vi "GetPodsStateData.vi"(11 "All Pods In":T17(array[cluster])) -> (2 "All Pod State Data":T18(array[cluster]), 3 "All Pods out":T17(array[cluster]))   [LabVIEW 2014]
uses:
  <vilib>/Rock Robotics/WPI/MotorControl/WPI_MotorControlDeviceRef.ctl
  <vilib>/Rock Robotics/WPI/MotorControl/WPI_MotorControlType.ctl
  <vilib>/Rock Robotics/SystemInterfaces/Typedef/FPGA_TypedefDigitalModule.ctl
  <vilib>/Rock Robotics/SystemInterfaces/DIO/FPGA_DIOPWMChannel.ctl
  <vilib>/Rock Robotics/WPI/PWM/WPI_PWMDeadband.ctl
  <vilib>/Rock Robotics/WPI/CAN/Jaguar/SubVIs/WPI_CANJaguar_ControlMode.ctl
  <vilib>/Rock Robotics/WPI/CAN/TalonSRX/WPI_CANTalonSRX_APIControlMode.ctl
  <vilib>/Rock Robotics/WPI/PWM/WPI_PWMTransform_ConPane.ctl
  <vilib>/Rock Robotics/WPI/AnalogChannel/WPI_AnalogChannelDevRef.ctl
  <vilib>/Rock Robotics/SystemInterfaces/Typedef/FPGA_TypedefAnalogModule.ctl
  <vilib>/Rock Robotics/SystemInterfaces/AI/FPGA_AIChannel.ctl
  <vilib>/Rock Robotics/WPI/Encoder/WPI_EncoderDevRef.ctl
  <vilib>/Rock Robotics/SystemInterfaces/Encoder/FPGA_EncoderIdx.ctl
  <vilib>/Rock Robotics/SystemInterfaces/Counter/FPGA_CounterCtrSystemIndex.ctl
  <vilib>/Rock Robotics/WPI/Encoder/WPI_EncoderType.ctl
  <vilib>/Rock Robotics/SystemInterfaces/Utilities/FPGA_UtilitiesRead LocalTime.vi
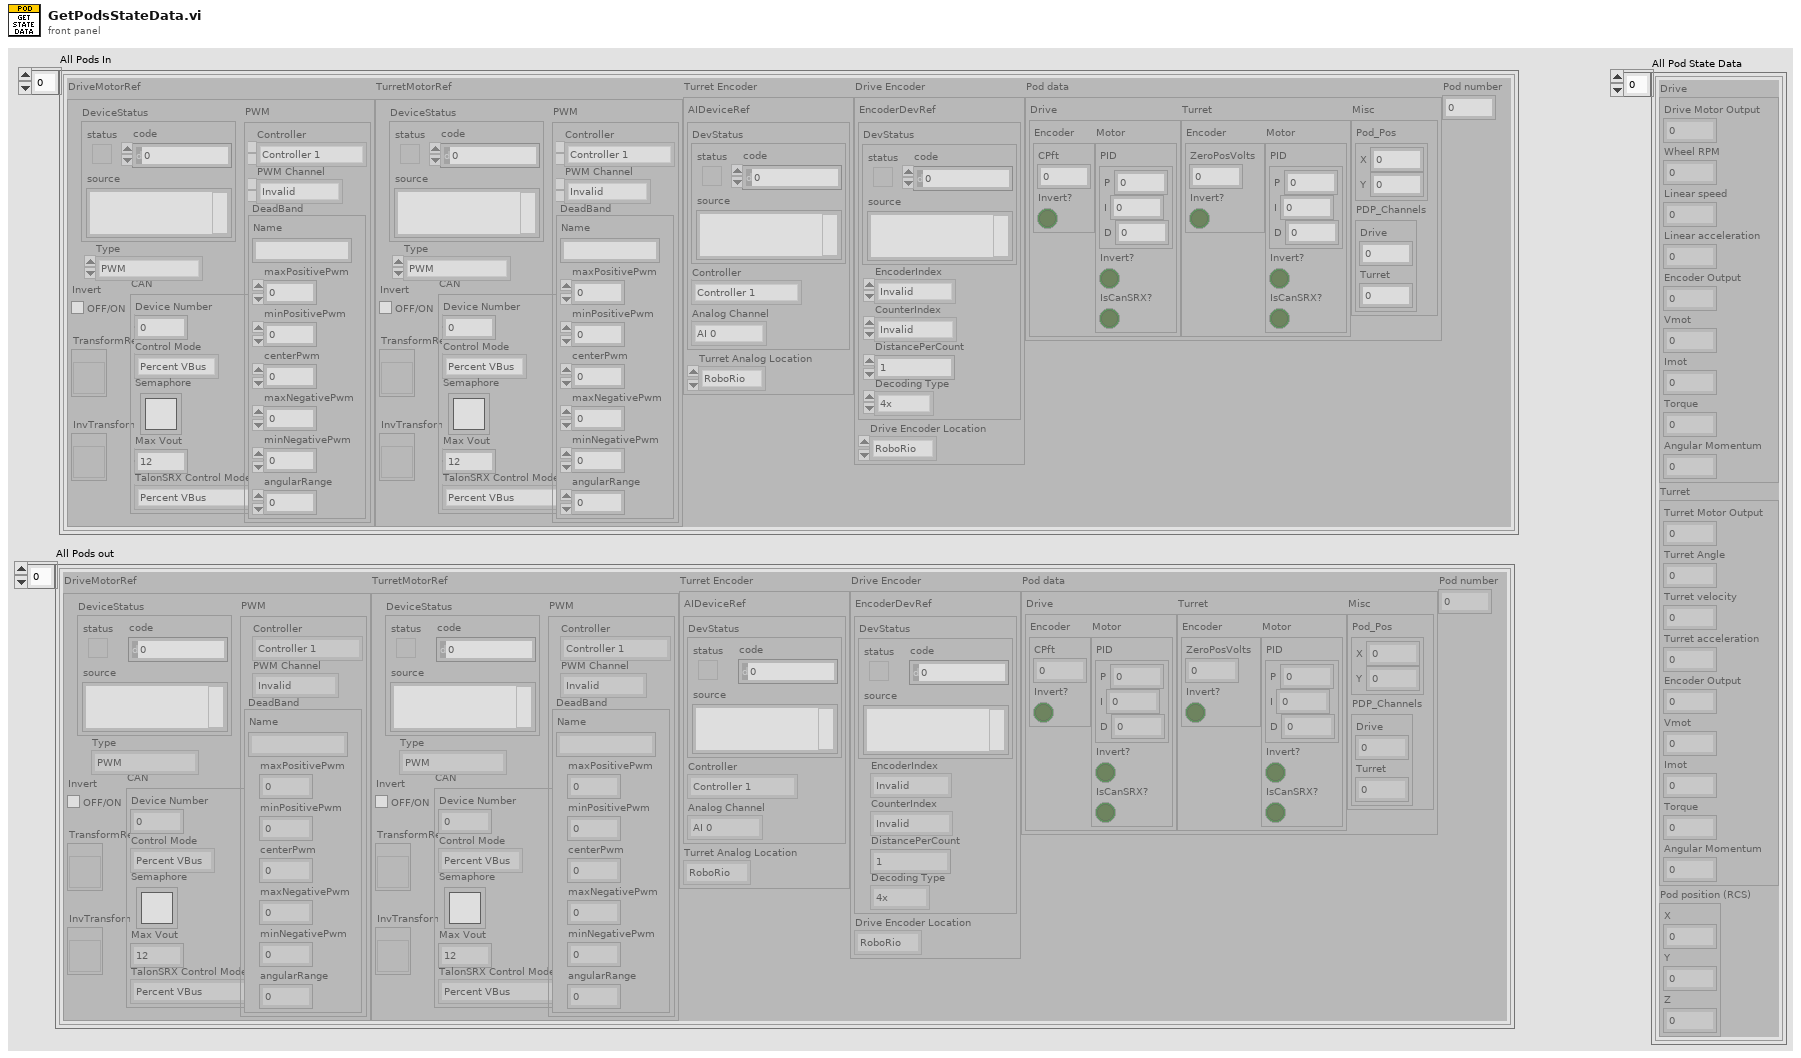
[diagram p1: front panel]
types:
  T1 = typedef "WPI_MotorControlDeviceRef.ctl" = cluster{"DeviceStatus":errorcluster, "Type":T2, "PWM":cluster{"Controller":T3, "PWM Channel":T4, "DeadBand":T5}, "CAN":cluster{"Device Number":u8, "Control Mode":T6, "Semaphore":T7, "Max Vout":dbl, "TalonSRX Control Mode":T8}, "Invert":bool, "TransformRef":T9, "InvTransformRef":T9}
  T2 = typedef "WPI_MotorControlType.ctl" = enum16{"PWM", "CAN", "CANTalonSRX"}
  T3 = typedef "FPGA_TypedefDigitalModule.ctl" = enum16{"Controller 1"}
  T4 = typedef "FPGA_DIOPWMChannel.ctl" = enum8{"PWM 0", "PWM 1", "PWM 2", "PWM 3", "PWM 4", "PWM 5", "PWM 6", "PWM 7", "PWM 8", "PWM 9", "PWM MXP 0", "PWM MXP 1", "PWM MXP 2", "PWM MXP 3", "PWM MXP 4", "PWM MXP 5", "PWM MXP 6", "PWM MXP 7", "PWM MXP 8", "PWM MXP 9", "Invalid"}
  T5 = typedef "WPI_PWMDeadband.ctl" = cluster{"Name":string, "maxPositivePwm":i32, "minPositivePwm":i32, "centerPwm":i32, "maxNegativePwm":i32, "minNegativePwm":i32, "angularRange":u16}
  T6 = typedef "WPI_CANJaguar_ControlMode.ctl" = enum8{"Percent VBus", "Current", "Speed", "Position", "Voltage"}
  T7 = typedef "Semaphore RefNum" = refnum<k1>
  T8 = typedef "WPI_CANTalonSRX_APIControlMode.ctl" = enum8{"Percent VBus", "Speed", "Position", "Slave", "Unchanged / Invalid"}
  T9 = typedef "WPI_PWMTransform_ConPane.ctl" = refnum<vi>
  T10 = typedef "WPI_AnalogChannelDevRef.ctl" = cluster{"DevStatus":errorcluster, "Controller":T11, "Analog Channel":T12}
  T11 = typedef "FPGA_TypedefAnalogModule.ctl" = enum16{"Controller 1"}
  T12 = typedef "FPGA_AIChannel.ctl" = enum8{"AI 0", "AI 1", "AI 2", "AI 3", "AI MXP 0", "AI MXP 1", "AI MXP 2", "AI MXP 3", "Invalid"}
  T13 = typedef "WPI_EncoderDevRef.ctl" = cluster{"DevStatus":errorcluster, "EncoderIndex":T14, "CounterIndex":T15, "DistancePerCount":dbl, "Decoding Type":T16}
  T14 = typedef "FPGA_EncoderIdx.ctl" = enum8{"Enc 0", "Enc 1", "Enc 2", "Enc 3", "Enc 4", "Enc 5", "Enc 6", "Enc 7", "Invalid"}
  T15 = typedef "FPGA_CounterCtrSystemIndex.ctl" = enum8{"Ctr 0", "Ctr 1", "Ctr 2", "Ctr 3", "Ctr 4", "Ctr 5", "Ctr 6", "Ctr 7", "Invalid"}
  T16 = typedef "WPI_EncoderType.ctl" = enum16{"1x", "2x", "4x"}
  T17 = cluster{"DriveMotorRef":T1, "TurretMotorRef":T1, "Turret Encoder":cluster{"AIDeviceRef":T10, "Turret Analog Location":enum16{"RoboRio", "Drive SRX", "Turret SRX"}}, "Drive Encoder":cluster{"EncoderDevRef":T13, "Drive Encoder Location":enum16{"RoboRio", "Drive SRX", "Turret SRX"}}, "Pod data":cluster{"Drive":cluster{"Encoder":cluster{"CPft":dbl, "Invert?":bool}, "Motor":cluster{"PID":cluster{"P":dbl, "I":dbl, "D":dbl}, "Invert?":bool, "IsCanSRX?":bool}}, "Turret":cluster{"Encoder":cluster{"ZeroPosVolts":dbl, "Invert?":bool}, "Motor":cluster{"PID":cluster{"P":dbl, "I":dbl, "D":dbl}, "Invert?":bool, "IsCanSRX?":bool}}, "Misc":cluster{"Pod_Pos":cluster{"X":dbl, "Y":dbl}, "PDP_Channels":cluster{"Drive":i32, "Turret":i32}}}, "Pod number":i32}[]
  T18 = cluster{"Drive":cluster{"Drive Motor Output":dbl, "Wheel RPM":dbl, "Linear speed":dbl, "Linear acceleration":dbl, "Encoder Output":dbl, "Vmot":dbl, "Imot":dbl, "Torque":dbl, "Angular Momentum":dbl}, "Turret":cluster{"Turret Motor Output":dbl, "Turret Angle":dbl, "Turret velocity":dbl, "Turret acceleration":dbl, "Encoder Output":dbl, "Vmot":dbl, "Imot":dbl, "Torque":dbl, "Angular Momentum":dbl}, "Pod position (RCS)":cluster{"X":dbl, "Y":dbl, "Z":dbl}}[]
  T19 = cluster{"Drive":cluster{"Drive Motor Output":dbl, "Wheel RPM":dbl, "Linear speed":dbl, "Linear acceleration":dbl, "Encoder Output":dbl, "Vmot":dbl, "Imot":dbl, "Torque":dbl, "Angular Momentum":dbl}, "Turret":cluster{"Turret Motor Output":dbl, "Turret Angle":dbl, "Turret velocity":dbl, "Turret acceleration":dbl, "Encoder Output":dbl, "Vmot":dbl, "Imot":dbl, "Torque":dbl, "Angular Momentum":dbl}, "Pod position (RCS)":cluster{"X":dbl, "Y":dbl, "Z":dbl}}
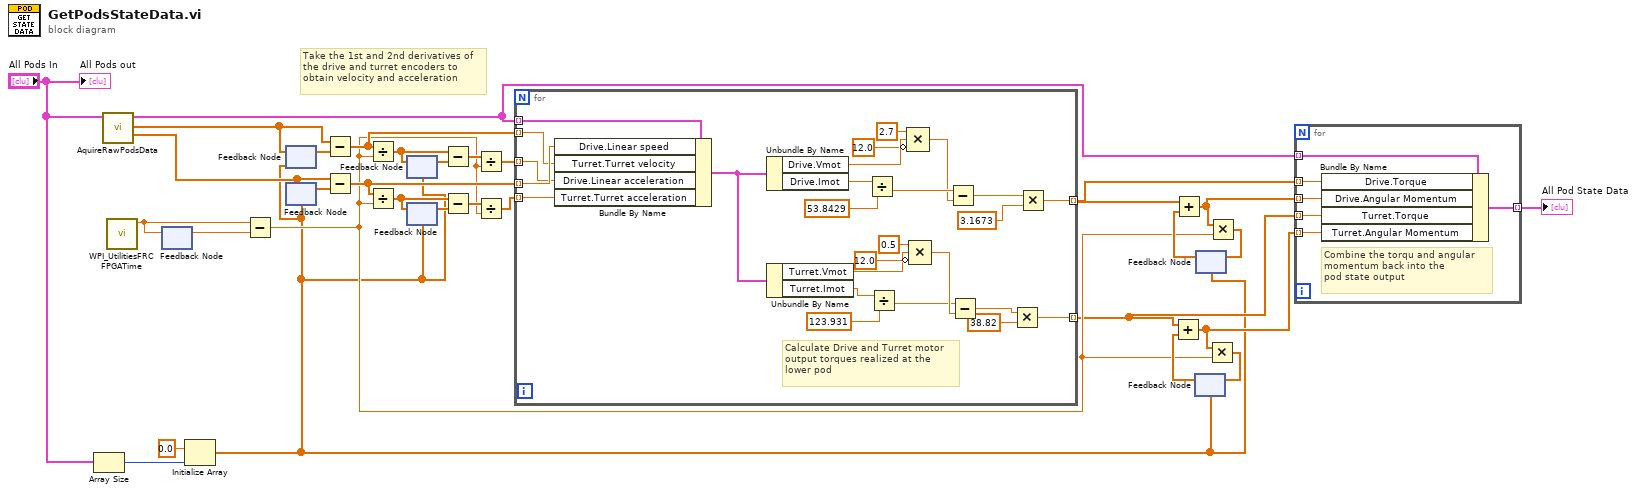
[diagram p0: block diagram]
diagram:
  # "Take the 1st and 2nd derivatives of\nthe drive and turret encoders to \nobtain velocity and acceleration"
  n1 = Array Size(array="All Pods In") -> (size(s)=w3:i32)
  n2 = call "AquireRawPodsData.vi"("All Pods In"="All Pods In") -> ("Turret Angles"=w31:dbl[], "Drive Encoder Outputs"=w28:dbl[], "Pods States"=w10:T18)  [unwired: 8 in]
  n3 = call <vilib>:"WPI_UtilitiesFRC FPGATime.vi"() -> ("FPGA Time"=w26:dbl)  [unwired: 10 in, 1 out]
  n4 = feedback #1() -> (w27:dbl)  [unwired: 1 in]
  n5 = feedback-in #1(w26) -> ()
  n6 = Initialize Array(0.0 ("element"), w3) -> (w1:dbl[])
  n7 = Subtract(x=w26, y=w27) -> (x-y=w11:dbl)
  n8 = feedback #2(w1) -> (w29:dbl[])
  n9 = feedback-in #2(w28) -> ()
  n10 = feedback-in #3(w31) -> ()
  n11 = feedback #3(w1) -> (w30:dbl[])
  n12 = Subtract(x=w28, y=w29) -> (x-y=w17:dbl[])
  n13 = Subtract(x=w31, y=w30) -> (x-y=w16:dbl[])
  n14 = Divide(x=w17, y=w11) -> (x/y=w20:dbl[])
  n15 = Divide(x=w16, y=w11) -> (x/y=w21:dbl[])
  n16 = feedback #4(w1) -> (w23:dbl[])
  n17 = feedback-in #4(w20) -> ()
  n18 = feedback #5(w1) -> (w22:dbl[])
  n19 = feedback-in #5(w21) -> ()
  n20 = Subtract(x=w20, y=w23) -> (x-y=w25:dbl[])
  n21 = Subtract(x=w21, y=w22) -> (x-y=w24:dbl[])
  n22 = Divide(x=w25, y=w11) -> (x/y=w18:dbl[])
  n23 = Divide(x=w24, y=w11) -> (x/y=w19:dbl[])
  n24 = for {
    tunnel: w19 -> [w53] mode=indexing
    tunnel: w18 -> [w54] mode=indexing
    tunnel: w10 -> [w57] mode=indexing
    tunnel: w17 -> [w55] mode=indexing
    tunnel: w16 -> [w56] mode=indexing
    tunnel: [w33] -> w9 mode=indexing
    tunnel: [w32] -> w7 mode=indexing
    # "Calculate Drive and Turret motor\noutput torques realized at the\nlower pod"
    n25 = Bundle By Name(cluster=w57, "Drive.Linear speed"=w56, "Turret.Turret velocity"=w55, "Drive.Linear acceleration"=w54, "Turret.Turret acceleration"=w53) -> (w38:T19)
    n26 = Unbundle By Name(w38) -> ("Drive.Vmot"=w50:dbl, "Drive.Imot"=w52:dbl)
    n27 = Unbundle By Name(w38) -> ("Turret.Vmot"=w41:dbl, "Turret.Imot"=w39:dbl)
    n28 = Divide(x=w52, y=53.8429) -> (x/y=w47:dbl)
    n29 = Divide(x=w39, y=123.931) -> (x/y=w44:dbl)
    n30 = Compound Arithmetic op=MULTIPLY(2.7 ("value"), w50, invert 12.0 ("value")) -> (w46:dbl)
    n31 = Compound Arithmetic op=MULTIPLY(0.5 ("value"), w41, invert 12.0 ("value")) -> (w45:dbl)
    n32 = Subtract(x=w47, y=w46) -> (x-y=w37:dbl)
    n33 = Subtract(x=w44, y=w45) -> (x-y=w35:dbl)
    n34 = Multiply(x=w35, y=38.82) -> (x*y=w32:dbl)
    n35 = Multiply(x=w37, y=3.1673) -> (x*y=w33:dbl)
  }
  n36 = feedback #6(w1) -> (w13:dbl[])
  n37 = Add(x=w7, y=w13) -> (x+y=w6:dbl[])
  n38 = feedback #7(w1) -> (w14:dbl[])
  n39 = Add(x=w9, y=w14) -> (x+y=w8:dbl[])
  n40 = Multiply(x=w6, y=w11) -> (x*y=w12:dbl[])
  n41 = feedback-in #6(w12) -> ()
  n42 = Multiply(x=w8, y=w11) -> (x*y=w15:dbl[])
  n43 = feedback-in #7(w15) -> ()
  n44 = for {
    tunnel: w10 -> [w63] mode=indexing
    tunnel: w9 -> [w60] mode=indexing
    tunnel: w8 -> [w59] mode=indexing
    tunnel: w7 -> [w61] mode=indexing
    tunnel: w6 -> [w62] mode=indexing
    tunnel: [w58] -> w5 mode=indexing
    # "Combine the torqu and angular\nmomentum back into the \npod state output"
    n45 = Bundle By Name(cluster=w63, "Drive.Torque"=w60, "Drive.Angular Momentum"=w59, "Turret.Torque"=w61, "Turret.Angular Momentum"=w62) -> (w58:T19)
  }
  "All Pod State Data" <- w5
  "All Pods out" <- "All Pods In"
